vi "SaveChunk.vi"(0 "Sensor2":dbl[](array[numeric]), 1 "All State":string[](array[string]), 5 "Sensor1":dbl[](array[numeric]), 7 "Path":path, 9 "Time(ms)":i64, 11 "Error In":errorcluster, 12 "Time interval":i64, 13 "all detect":string[](array[string])) -> (4 "Time (ms) out":i64, 15 "Error Out":errorcluster)   [LabVIEW 2016]
doc: "save chunk of data. The chunk is the maximum number of elements s.t. the number is equal from both sensors"
panel:
  out "transposed array":dbl[][](array[numeric])
  out "string array":string[][](array[string])
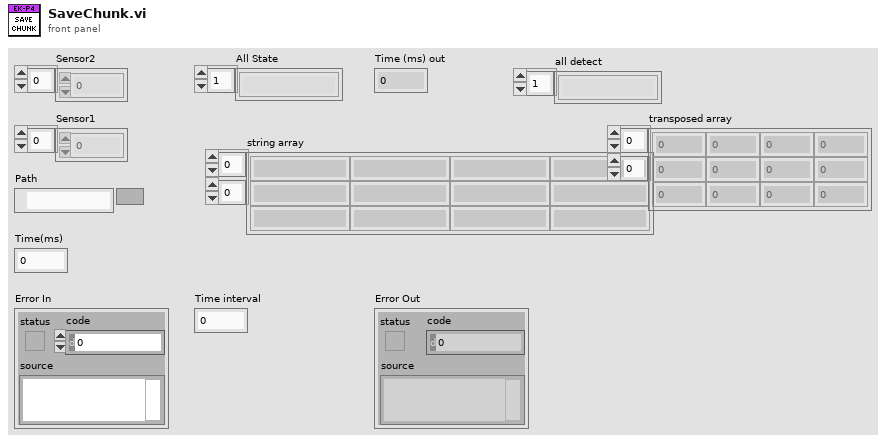
[diagram p1: front panel]
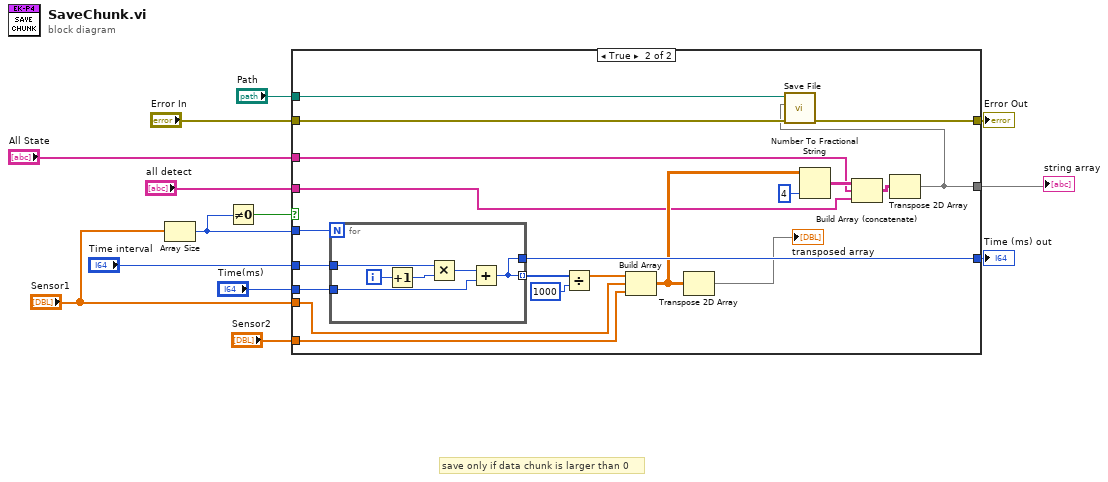
[diagram p0: block diagram]
diagram:
  # "save only if data chunk is larger than 0"
  n1 = Array Size(array="Sensor1") -> (size(s)=w9:i32)
  n2 = Not Equal To 0?(x=w9) -> (x != 0?=w11:bool)
  n3 = case shown="True" w11 {
    tunnel: "Time(ms)" -> [w15 w31]
    tunnel: "Sensor1" -> [_ w34]
    tunnel: [w15 w32] -> w10
    tunnel: w9 -> [_ w33]
    tunnel: "Sensor2" -> [_ w30]
    tunnel: [w14 w29] -> w7
    tunnel: "Error In" -> [w14 w28]
    tunnel: "Path" -> [_ w27]
    tunnel: "Time interval" -> [_ w26]
    tunnel: "All State" -> [_ w21]
    tunnel: [_ w17] -> w2
    tunnel: "all detect" -> [_ w16]
    frame False {
    }
    frame True {
      n4 = for {
        N: w33 -> [_]
        tunnel: w26 -> [w37]
        tunnel: w31 -> [w36]
        tunnel: [w39] -> w35 mode=indexing
        tunnel: [w39] -> w32
        i -> [w41]
        n5 = Increment(x=w41) -> (x+1=w38:i32)
        n6 = Multiply(x=w37, y=w38) -> (x*y=w40:i64)
        n7 = Add(x=w40, y=w36) -> (x+y=w39:i64)
      }
      n8 = Divide(x=w35, y=1000) -> (x/y=w25:dbl[])
      n9 = Build Array(w25, w34, w30) -> (w18:dbl[][])
      n10 = Transpose 2D Array(2D array=w18) -> (transposed array=→"transposed array":dbl[][])
      n11 = Number To Fractional String(number=w18, precision (6)=i16 4 ("width (-)")) -> (F-format string=w22:string[][])  [unwired: 2 in]
      n12 = Build Array (concatenate)(w22, w21, w16) -> (w20:string[][])
      n13 = Transpose 2D Array(2D array=w20) -> (transposed array=w17:string[][])
      n14 = call "Save File.vi"("error in (no error)"=w28, "Array"=w17, "Path"=w27) -> ("error out"=w29:errorcluster)  [unwired: 8 in]
    }
  }
  "Time (ms) out" <- w10
  "Error Out" <- w7
  "string array" <- w2
